vi "Alliance Color.vi"() -> (0 "Alliance Color":u32(colorbox)=16714752)   [LabVIEW 2016]
uses:
  <vilib>/Rock Robotics/Network Tables/NT Read String.vi
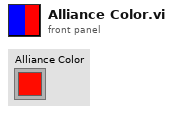
[diagram p1: front panel]
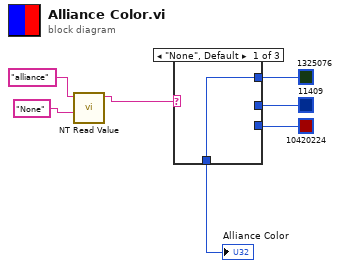
[diagram p0: block diagram]
diagram:
  n1 = call-poly <vilib>:"NT Read Value.vi"("Default Value"="None", "Name"="alliance") -> ("String"=w5:string)  [unwired: 8 in, 1 out]
  n2 = case shown="\"None\", Default" w5 {
    tunnel: [w8 w9 w10] -> w4
    tunnel: u32 1325076 -> [w8 _ _]
    tunnel: u32 11409 -> [_ w9 _]
    tunnel: u32 10420224 -> [_ _ w10]
    frame "None", Default {
    }
    frame "Blue" {
    }
    frame "Red" {
    }
  }
  "Alliance Color" <- w4
